vi "Test Test Finder Do Not Ignore Inherited Methods.vi"(8 "error in (no error)":errorcluster, 11 "Test Finder In":refnum<class "Finder Test.lvclass">) -> (0 "error out":errorcluster, 3 "Test Finder Out":refnum<class "Finder Test.lvclass">)   [LabVIEW 2020, in "LUnit Tests.lvlib" / "Finder Test.lvclass"]
uses:
  Finder Test.lvclass
  source/Framework/Helper Classes/Test Finder/Test Finder.lvclass
  Test Dummys/Descending Test Test Case/Descending Test Test Case.lvclass
  16ef78da-0e29-4b5c-aa18-7c402dca1234.vi
  source/Framework/Test Suite/LUnit Test Suite.lvclass
  source/Framework/Test Case/LUnit Test Case.lvclass
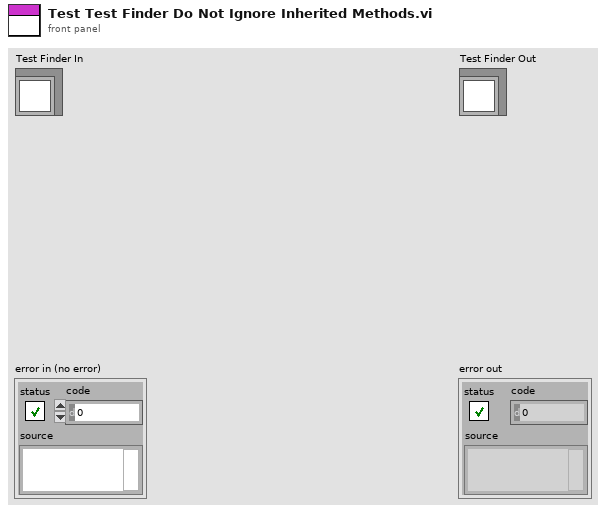
[diagram p1: front panel]
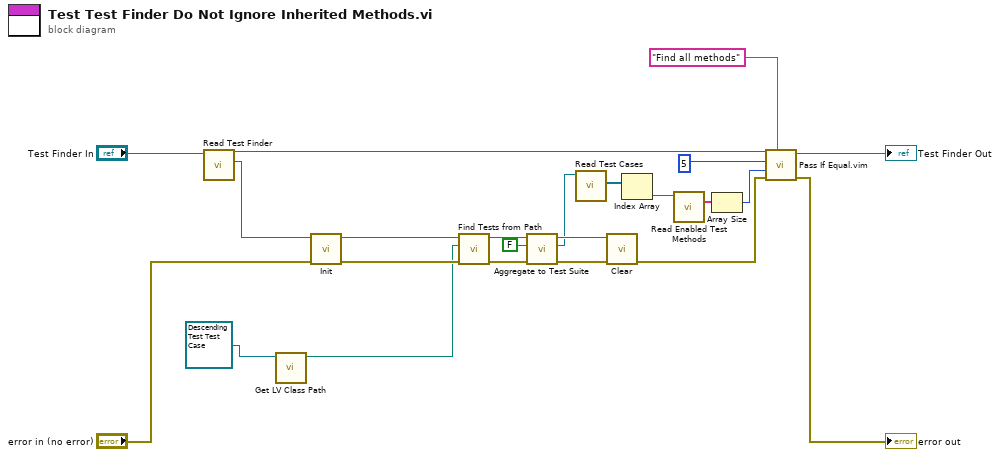
[diagram p0: block diagram]
diagram:
  n1 = call "Read Test Finder.vi"("Test Finder In"="Test Finder In") -> ("Test Finder.lvclass"=w22:refnum<class "Test Finder.lvclass">, "Test Finder Out"=w12:refnum<class "Finder Test.lvclass">)  [unwired: 8 in, 1 out]
  n2 = call <vilib>:"Get LV Class Path.vi"("object"=refnum<class "Descending Test Test Case.lvclass"> refnum ("Descending Test Test Case.lvclass")) -> ("class path"=w18:path)  [unwired: 9 in, 1 out]
  n3 = call-dynamic "Init.vi"("error in (no error)"="error in (no error)", "Test Finder in"=w22) -> ("error out"=w20:errorcluster, "Test Finder out"=w21:refnum<class "Test Finder.lvclass">)  [unwired: 8 in]
  n4 = call-dynamic "Find Tests from Path.vi"("error in (no error)"=w20, "Project or Class Path"=w18, "Test Case Finder In"=w21) -> ("error out"=w15:errorcluster, "Test Case Finder Out"=w17:refnum<class "Test Finder.lvclass">)  [unwired: 7 in]
  n5 = call "Aggregate to Test Suite.vi"("error in (no error)"=w15, "Ignore Inherited Tests?"=FALSE, "Test Finder In"=w17) -> ("error out"=w14:errorcluster, "Test Suite"=w5:refnum<class "LUnit Test Suite.lvclass">, "Test Finder Out"=w16:refnum<class "Test Finder.lvclass">)  [unwired: 6 in]
  n6 = call "Read Test Cases.vi"("Test Suite In"=w5) -> ("Test Cases"=w4:refnum<class "LUnit Test Case.lvclass">[])  [unwired: 9 in, 1 out]
  n7 = call "Clear.vi"("error in (no error)"=w14, "Test Finder in"=w16) -> ("error out"=w10:errorcluster)  [unwired: 8 in, 1 out]
  n8 = Index Array(array=w4) -> (element=w3:refnum<class "LUnit Test Case.lvclass">)  [unwired: 1 in]
  n9 = call "Read Enabled Test Methods.vi"("LUnit Test Case In"=w3) -> ("Names"=w2:string[])  [unwired: 8 in, 2 out]
  n10 = Array Size(array=w2) -> (size(s)=w1:i32)
  n11 = call "Pass If Equal.vim"("Description"="Find all methods", "error in (no error)"=w10, "Actual"=w1, "Expected"=5 ("x"), "LUnit Test Case In"=w12) -> ("error out"=→"error out":errorcluster, "LUnit Test Case Out"=→"Test Finder Out":refnum<class "Finder Test.lvclass">)  [unwired: 5 in]
